vi "ma_sml_Peak Rough Search Indices.vi"   [LabVIEW 2020, in "NI_MAPro.lvlib"]
uses:
  NI_MAPro.lvlib
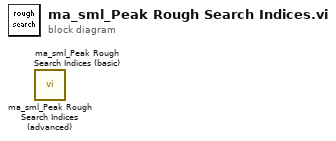
[diagram p0: block diagram]
diagram:
  n1 = call "ma_sml_Peak Rough Search Indices (advanced).vi"() -> ()  [unwired: 5 in, 1 out]
  n2 = call "ma_sml_Peak Rough Search Indices (basic).vi"() -> ()  [unwired: 5 in, 1 out]
